vi "Create submenu.vi"(6 "after item":string, 7 "owning menu tag":string, 8 "error in (no error)":errorcluster, 10 "tag in":string, 11 "Menu in":refnum<k9>) -> (0 "error out":errorcluster, 2 "tag out":string, 3 "Menu out":refnum<k9>)   [LabVIEW 2020, in "Menu From Cluster.lvlib"]
uses:
  <vilib>/JDP Science/JDP Science Common Utilities/Shortcut Menu Tools/Menu From Cluster.lvlib
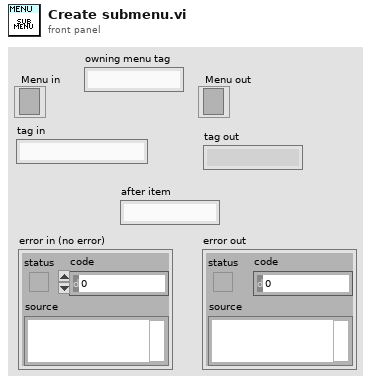
[diagram p1: front panel]
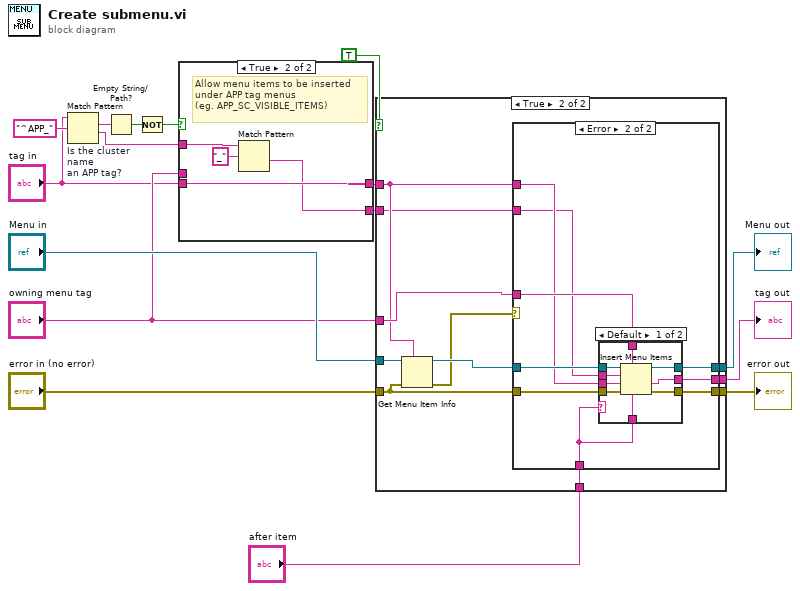
[diagram p0: block diagram]
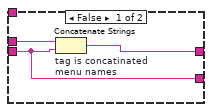
[diagram p2: hidden frame]
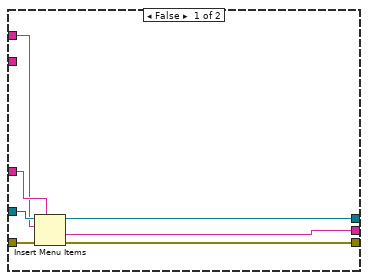
[diagram p3: hidden frame]
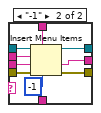
[diagram p5: hidden frame]
diagram:
  n1 = Match Pattern "Is the cluster\nname\nan APP tag?"(string="tag in", regular expression="^APP_") -> (match substring=w9:string, after substring=w3:string)  [unwired: 1 in, 2 out]
  n2 = Empty String/Path?(string/path=w9) -> (empty?=w16:bool)
  n3 = Not(x=w16) -> (.not. x?=w8:bool)
  n4 = case shown="True" w8 {
    tunnel: "owning menu tag" -> [w19 _]
    tunnel: "tag in" -> [w17 w23]
    tunnel: [w18 w23] -> w5
    tunnel: [w17 w20] -> w4
    tunnel: w3 -> [_ w22]
    frame False {
      n5 = Concatenate Strings "tag is concatinated \nmenu names"(w19, w17) -> (w18:string)
    }
    frame True {
      # "Allow menu items to be inserted\nunder APP tag menus\n(eg. APP_SC_VISIBLE_ITEMS)"
      n6 = Match Pattern(string=w22, regular expression="_") -> (after substring=w20:string)  [unwired: 1 in, 3 out]
    }
  }
  n7 = case shown="True" TRUE {
    tunnel: "Menu in" -> [w30 w41]
    tunnel: [w29 w35] -> w11
    tunnel: "owning menu tag" -> [w28 w39]
    tunnel: [w27 w36] -> w12
    tunnel: "error in (no error)" -> [w26 w34]
    tunnel: [w25 w37] -> w13
    tunnel: w5 -> [w24 w38]
    tunnel: w4 -> [_ w33]
    tunnel: "after item" -> [_ w31]
    frame False {
      n8 = Insert Menu Items(5:w28, 6:w26, 8:w24, 9:w30) -> (0:w25:errorcluster, 1:w27:string, 3:w29:refnum<k9>)  [unwired: 1 in, 1 out]
    }
    frame True {
      n9 = Get Menu Item Info(7:w38, 8:w34, 11:w41) -> (0:w32:errorcluster, 3:w40:refnum<k9>)  [unwired: 5 out]
      n10 = case shown="Error" w32 {
        tunnel: w40 -> [w44 w53]
        tunnel: w39 -> [_ w48]
        tunnel: w38 -> [w43 w47]
        tunnel: w34 -> [w42 w52]
        tunnel: [w42 w51] -> w37
        tunnel: [w43 w50] -> w36
        tunnel: [w44 w49] -> w35
        tunnel: w33 -> [_ w46]
        tunnel: w31 -> [_ w45]
        frame No Error {
          # "Already exists"
        }
        frame Error {
          n11 = case shown="Default" w45 {
            tunnel: w53 -> [w62 w71]
            tunnel: w52 -> [w61 w70]
            tunnel: [w60 w69] -> w51
            tunnel: [w59 w68] -> w50
            tunnel: [w58 w67] -> w49
            tunnel: w48 -> [w57 w66]
            tunnel: w47 -> [w56 w65]
            tunnel: w46 -> [w55 w64]
            tunnel: w45 -> [w54 _]
            frame Default {
              n12 = Insert Menu Items(4:w54, 5:w57, 6:w61, 7:w56, 8:w55, 9:w62) -> (0:w60:errorcluster, 1:w59:string, 3:w58:refnum<k9>)
            }
            frame "-1" {
              n13 = Insert Menu Items(4:-1, 5:w66, 6:w70, 7:w65, 8:w64, 9:w71) -> (0:w69:errorcluster, 1:w68:string, 3:w67:refnum<k9>)
            }
          }
        }
      }
    }
  }
  "error out" <- w13
  "tag out" <- w12
  "Menu out" <- w11
